vi "Run.vi"(8 "error in (no error)":errorcluster, 11 "Parameter In":refnum<class "Parameter.lvclass">) -> (0 "error out":errorcluster, 1 "Done?":bool, 2 "Results":T1(array[cluster]), 3 "Parameter Out":refnum<class "Parameter.lvclass">)   [LabVIEW 2020, in "Parameter.lvclass"]
uses:
  Parameter.lvclass
  Parameter.lvclass/Parameter.ctl
  <vilib>/Astemes/LUnit/Test Case.lvclass
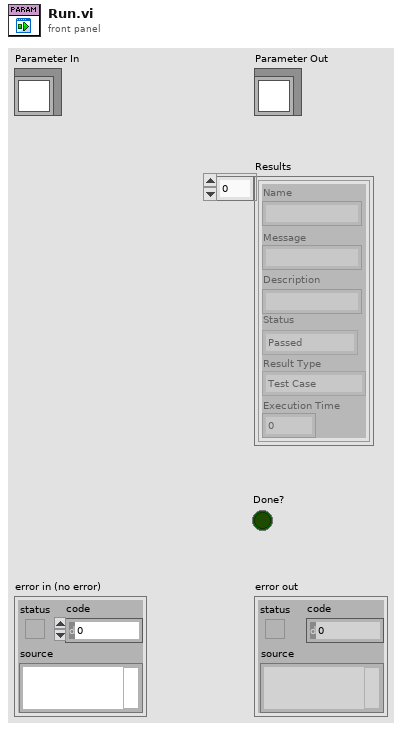
[diagram p1: front panel]
types:
  T1 = cluster{"Name":string, "Message":string, "Description":string, "Status":enum16{"", "Passed", "Failed", "Error", "Skipped", "Setup Error", "Broken", "Teardown Error"}, "Result Type":enum16{"Test Case", "Test Suite", "Test Run", "Pass", "Fail", "Skip", "Pass if", "Fail if", "Pass if Error", "Fail if Error", "Pass if Equal", "Fail if Equal"}, "Execution Time":dbl}[]
  T2 = cluster{"Name":string, "Message":string, "Description":string, "Status":enum16{"", "Passed", "Failed", "Error", "Skipped", "Setup Error", "Broken", "Teardown Error"}, "Result Type":enum16{"Test Case", "Test Suite", "Test Run", "Pass", "Fail", "Skip", "Pass if", "Fail if", "Pass if Error", "Fail if Error", "Pass if Equal", "Fail if Equal"}, "Execution Time":dbl}
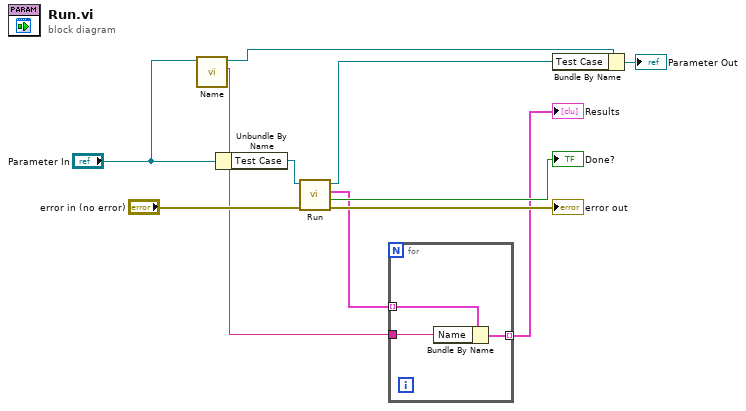
[diagram p0: block diagram]
diagram:
  n1 = call-dynamic "Name.vi"("Runnable in"="Parameter In") -> ("Name"=w2:string, "Runnable out"=w3:refnum<class "Parameter.lvclass">)  [unwired: 8 in, 1 out]
  n2 = Unbundle By Name("Parameter In") -> ("Test Case"=w9:refnum<class "Test Case.lvclass">)
  n3 = call-dynamic "Run.vi"("error in (no error)"="error in (no error)", "LUnit Test Case In"=w9) -> ("error out"=→"error out":errorcluster, "Done?"=→"Done?":bool, "Results"=w5:T1, "LUnit Test Case Out"=w6:refnum<class "Test Case.lvclass">)  [unwired: 6 in]
  n4 = for {
    tunnel: w5 -> [w14] mode=indexing
    tunnel: w2 -> [w13]
    tunnel: [w12] -> w1 mode=indexing
    n5 = Bundle By Name(cluster=w14, "Name"=w13) -> (w12:T2)
  }
  "Results" <- w1
  n6 = Bundle By Name(cluster=w3, "Test Case"=w6) -> (→"Parameter Out":refnum<class "Parameter.lvclass">)
